vi "Obtain Report.vi"(0 "Session Handle in":T2, 11 "error in (no error)":errorcluster) -> (4 "Session Handle out":T2, 8 "Report":T1, 15 "error out":errorcluster)   [LabVIEW 2020, in "TSS.lvlib" / "Execution.lvclass"]
uses:
  Execution.lvclass
  Typedefs/Session Handle.ctl
  Report/Typedefs/Session Handle.ctl
  Report/Report.lvclass
  Get Engine.vi
  Engine/Engine.lvclass
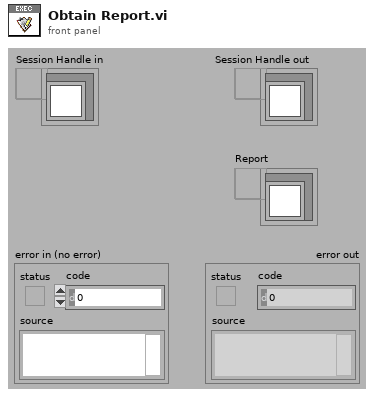
[diagram p1: front panel]
types:
  T1 = typedef "TSS.lvlib/Report.lvclass/Session Handle.ctl" = refnum<data-value>
  T2 = typedef "TSS.lvlib/Execution.lvclass/Session Handle.ctl" = refnum<data-value>
  T3 = typedef "TSS.lvlib/Engine.lvclass/Session Handle.ctl" = refnum<data-value>
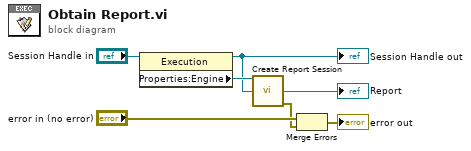
[diagram p0: block diagram]
diagram:
  n1 = property class="Execution"(reference="Session Handle in") -> (reference out=w4:T2, "Properties:Engine"=w5:T3)  [unwired: 1 in, 1 out]
  "Session Handle out" <- w4
  n2 = call "Create Report Session.vi"("Session Handle in"=w5, "Execution"=w4) -> ("Report"=→"Report":T1, "error out"=w2:errorcluster)  [unwired: 11 in, 1 out]
  n3 = Merge Errors("error in (no error)", w2) -> (→"error out":errorcluster)
